vi "Write N.vi"(5 "N":refnum<class "Tunnel.lvclass">, 9 "ForLoop in":refnum<class "ForLoop.lvclass">) -> (3 "ForLoop out":refnum<class "ForLoop.lvclass">)   [LabVIEW 2014, in "ForLoop.lvclass"]
uses:
  ForLoop.lvclass
  Tunnel/Tunnel.lvclass
  ForLoop.lvclass/ForLoop.ctl
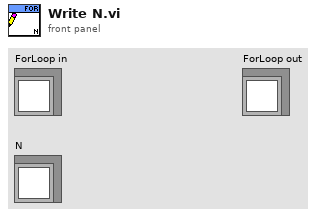
[diagram p1: front panel]
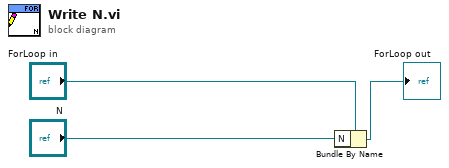
[diagram p0: block diagram]
diagram:
  n1 = Bundle By Name(cluster="ForLoop in", "N"="N") -> (→"ForLoop out":refnum<class "ForLoop.lvclass">)
